vi "Remaining_timestamp.vi"(7 "Time period target":dbl caption="Time period target [s]", 11 "Error in":errorcluster caption="Error in (no error)", 12 "Start time in":timestamp caption="Start time in (0: init)") -> (8 "Remaining time":dbl caption="Remaining time [s]", 10 "Elapsed time":dbl caption="Elapsed time [s]", 13 "Now":timestamp, 14 "Start time out":timestamp, 15 "Error out":errorcluster)   [LabVIEW 2017, in "GPTiming.lvlib"]
doc: "Calculates <B>Remaining time</B> of <B>Time period target</B> since <B>Start time in</B>.\n\n<B>Start time in</B> will be returned in <B>Start time out</B>. Set <B>Start time in</B> to a default-valued zero timestamp (or leave it unwired) to get the current time returned in <B>Start time out</B> instead. <B>Now</B> will always be the current time.\n\nThis VI counts time with timestamps and will be able to count with ms accuracy until the year 3000 (the current maximum year of a LabVIEW timestamp). Using timestamps consume about three times as many CPU-cycles as using the tick counter (it's still measured in nanoseconds), but the timing range is increased tremendously. <B>Remaining time</B> will be latched at 0 when the remaining time runs out. <B>Elapsed time</B> will continue counting up past the remaining time running out, thus you can use this output to see how late you were if you overshoot the <B>Time period target</B>.\n\nThis VI is inlined. <B>Error in</B> is wired straight through to <B>Error out</B> to enable optional dataflow dependency (offering control of when <B>Now</B> is).\n\nSteen Schmidt\nGPower\n6/12 2013"
uses:
  GPTiming.lvlib
panel:
  # "Copyright © 2013\nGPower\nSee enclosed license file for terms and conditions"
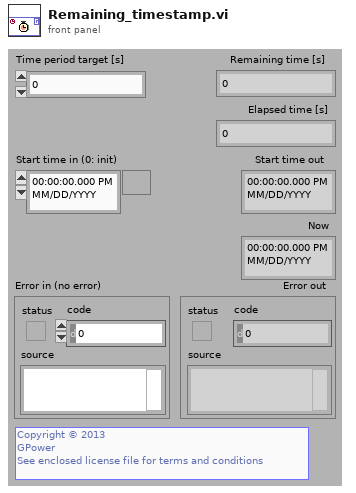
[diagram p1: front panel]
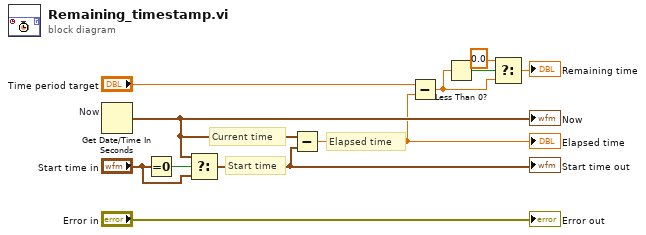
[diagram p0: block diagram]
diagram:
  # "Elapsed time"
  # "Current time"
  # "Start time"
  n1 = Get Date/Time In Seconds "Now"() -> (seconds since 1Jan1904=w2:timestamp)
  "Now" <- w2
  n2 = Equal To 0?(x="Start time in") -> (x = 0?=w10:bool)
  n3 = Select(t=w2, s=w10, f="Start time in") -> (s? t:f=w8:timestamp)
  "Start time out" <- w8
  n4 = Subtract(x=w2, y=w8) -> (x-y=w1:dbl)
  "Elapsed time" <- w1
  n5 = Subtract(x="Time period target", y=w1) -> (x-y=w4:dbl)
  n6 = Less Than 0?(x=w4) -> (x < 0?=w5:bool)
  n7 = Select(t=0.0, s=w5, f=w4) -> (s? t:f=→"Remaining time":dbl)
  "Error out" <- "Error in"
